vi "AIn.vi"(2 "Length":u8, 3 "1st ch#":u8) -> (0 "Ain[]":dbl[](array[numeric]) format="%.2f", 1 "Ains[]":i32[](array[numeric]))   [LabVIEW 2011]
uses:
  Globals/DynaGlbs.vi
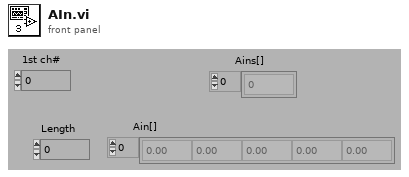
[diagram p1: front panel]
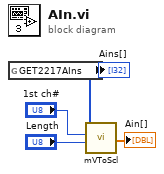
[diagram p0: block diagram]
diagram:
  n1 = global read "DynaGlbs.vi" "GET2217AIns"() -> (w1:i32[])
  "Ains[]" <- w1
  n2 = call "mVToScl.vi"("Length"="Length", "1st ch#"="1st ch#", "Ain[]"=w1) -> ("Scale"=→"Ain[]":dbl[])  [unwired: 3 in]
